vi "GetNumberOfItems.vi"(0 "reference in":refnum<class "Box.lvclass">, 5 "Error In":errorcluster) -> (14 "reference out":refnum<class "Box.lvclass">, 16 "ItemsInside":T1, 19 "Error Out":errorcluster)   [LabVIEW 2024, in "Box.lvclass"]
doc: "Get number of items inside the box recursively"
uses:
  Box.lvclass
  Items Inside Map.ctl
  Component_interface/Component.lvclass
panel:
  # "Connector Pane"
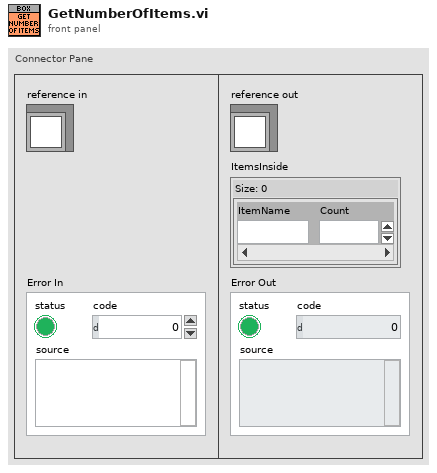
[diagram p1: front panel]
types:
  T1 = typedef "Items Inside Map.ctl" = map{string, u64}
  T2 = typedef "Box.lvclass/ObjectAttributes.ctl" = cluster{"Components":refnum<class "Component.lvclass">[], "ItemsInside":T1}
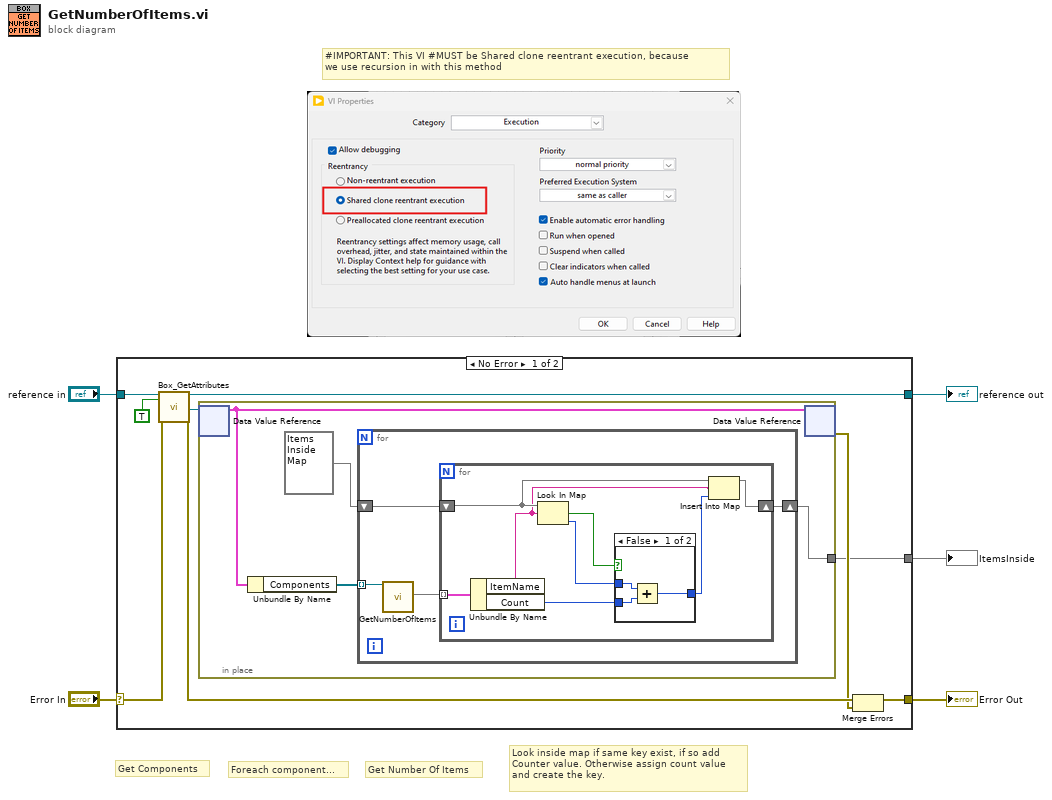
[diagram p0: block diagram]
diagram:
  # "Look inside map if same key exist, if so add\nCounter value. Otherwise assign count value\nand create the key."
  # "Get Number Of Items"
  # "Foreach component..."
  # "Get Components"
  # "#IMPORTANT: This VI #MUST be Shared clone reentrant execution, because\nwe use recursion in with this method"
  n1 = case shown="No Error" "Error In" {
    selector: "Error In" -> [w13 w36]
    tunnel: [w11 w36] -> w4
    tunnel: [w12 w35] -> w2
    tunnel: "reference in" -> [w14 w35]
    tunnel: [w6 _] -> w1
    frame No Error {
      n2 = call "Box_GetAttributes.vi"("reference in"=w14, "OnlyGetDvrReference(False)"=TRUE, "Error In"=w13) -> ("reference out"=w12:refnum<class "Box.lvclass">, "DataRef"=w10:refnum<data-value>, "Error Out"=w8:errorcluster)  [unwired: 13 in, 1 out]
      n3 = in-place {
        in-place-border: [w15] -> w6
        n4 = in-place-dvr #1(w10) -> (w18:T2)  [unwired: 1 out]
        n5 = Unbundle By Name(w18) -> ("Components"=w17:refnum<class "Component.lvclass">[])
        n6 = for {
          tunnel: w17 -> [w22] mode=indexing
          shift-right: [w19] -> w15
          shift-left: T1 {} ("ItemsInside") -> [w20]
          n7 = call-dynamic "GetNumberOfItems.vi"("object in"=w22) -> ("ItemsInside"=w21:T1)  [unwired: 16 in, 2 out]
          n8 = for {
            tunnel: w21 -> [w30] mode=indexing
            shift-right: [w29] -> w19
            shift-left: w20 -> [w28]
            n9 = Unbundle By Name(w30) -> ("ItemName"=w24:string, "Count"=w26:u64)
            n10 = Look In Map(map=w28, key=w24) -> (key not found?=w27:bool, value=w23:u64)  [unwired: 1 in]
            n11 = case shown="False" w27 {
              tunnel: w26 -> [w32 w34]
              tunnel: [w31 w34] -> w25
              tunnel: w23 -> [w33 _]
              frame False {
                n12 = Add(x=w33, y=w32) -> (x+y=w31:u64)
              }
              frame True {
              }
            }
            n13 = Insert Into Map(map in=w28, key=w24, value=w25) -> (map out=w29:T1)  [unwired: 2 out]
          }
        }
        n14 = in-place-dvr #1(w18) -> (w7:errorcluster)  [unwired: 1 out]
      }
      n15 = Merge Errors(w8, w7) -> (w11:errorcluster)
    }
    frame Error {
    }
  }
  "Error Out" <- w4
  "reference out" <- w2
  "ItemsInside" <- w1
